vi "搜索字符串 (子VI).vi"(11 "read buffer":string) -> (3 "数组":string[](array[string]))   [LabVIEW 2013]
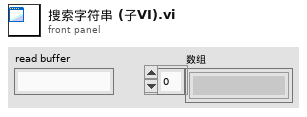
[diagram p1: front panel]
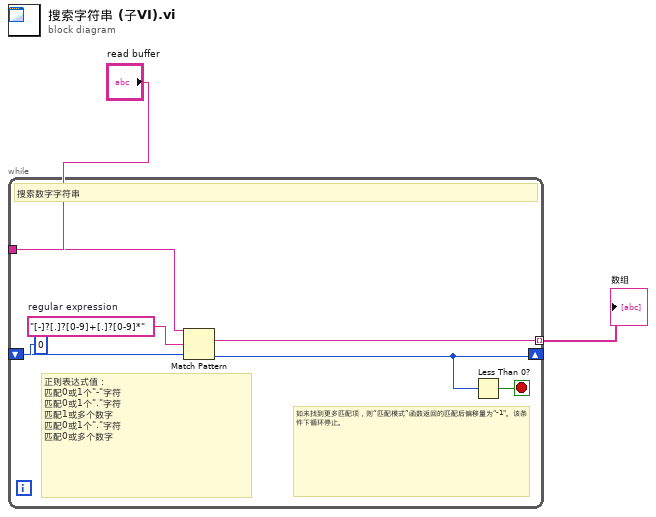
[diagram p0: block diagram]
diagram:
  n1 = while {
    tunnel: "read buffer" -> [w9]
    shift-left: 0 -> [w7]
    shift-right: [w6] -> _
    tunnel: [w4] -> w3 mode=indexing
    stop <- w8 stop-if-true
    w5 = "[-]?[.]?[0-9]+[.]?[0-9]*"  # regular expression
    # "如未找到更多匹配项，则“匹配模式”函数返回的匹配后偏移量为\"-1\"。该条件下循环停止。"
    # "正则表达式值：\n匹配0或1个\"-\"字符\n匹配0或1个\".\"字符\n匹配1或多个数字\n匹配0或1个\".\"字符\n匹配0或多个数字"
    # "搜索数字字符串"
    n2 = Match Pattern(string=w9, regular expression=w5, offset (0)=w7) -> (match substring=w4:string, offset past match=w6:i32)  [unwired: 2 out]
    n3 = Less Than 0?(x=w6) -> (x < 0?=w8:bool)
  }
  "数组" <- w3
